vi "SPI API - SPI Simulation.vi"() -> ()   [LabVIEW 2015]
uses:
  Controls/Timing Characteristics.ctl
  Controls/Digital Data.ctl
  <vilib>/rvi/DesktopExecutionNode/Execution/niFpgaDEN_Execute.vi
  <vilib>/rvi/DesktopExecutionNode/DesktopExecutionNode.xnode
panel:
  out "Data 8":u64
  out "Data 7":u64
  out "Data 6":u64
  out "Data 5":u64
  out "Slave Response":u64
  out "Data To Slave":u64 format="%b"
  out "Timing Characteristics":T1 {"tCL (ns)" format="%#_4g"; "tCH (ns)" format="%#_4g"; "tCP (ns)" format="%#_4g"; "tCSS (ns)" format="%#_4g"; "tCSH (ns)" format="%#_4g"; "tCSW (ns)" format="%#_4g"; "Actual Sample Rate (Hz)" format="%_4p"; "SCLK Frequency (Hz)" format="%#.2p"}
  in  "Pause":bool
  in  "SPI PHY Settings":T2={"Divide Value"=10, "Transfer Length (bits)"=24, "CS Asserted Polarity"=FALSE, "Clock Polarity (CPOL)"=FALSE, "Clock Phase (CPHA)"=FALSE, "Lengthen MISO Setup"=FALSE, "Direction Change Bit"=0, "MOSI Starts as Output"=FALSE, "Tristatable MOSI"=FALSE}
  out "Digital Data":digitalwaveform(graph)
  in  "Data To Slave":u64
  in  "Stop":bool
  # "Operating Instructions\n1. For this VI to work, the FPGA must be in Simulation Mode.\n2. Run the VI and change the 'SPI PHY Settings' and 'Data To Slave' controls to change the SPI Output.\n3. While changing the settings, view the timing characteristics of the signal on the right side of the graph."
  # "Typical Timing Diagram"
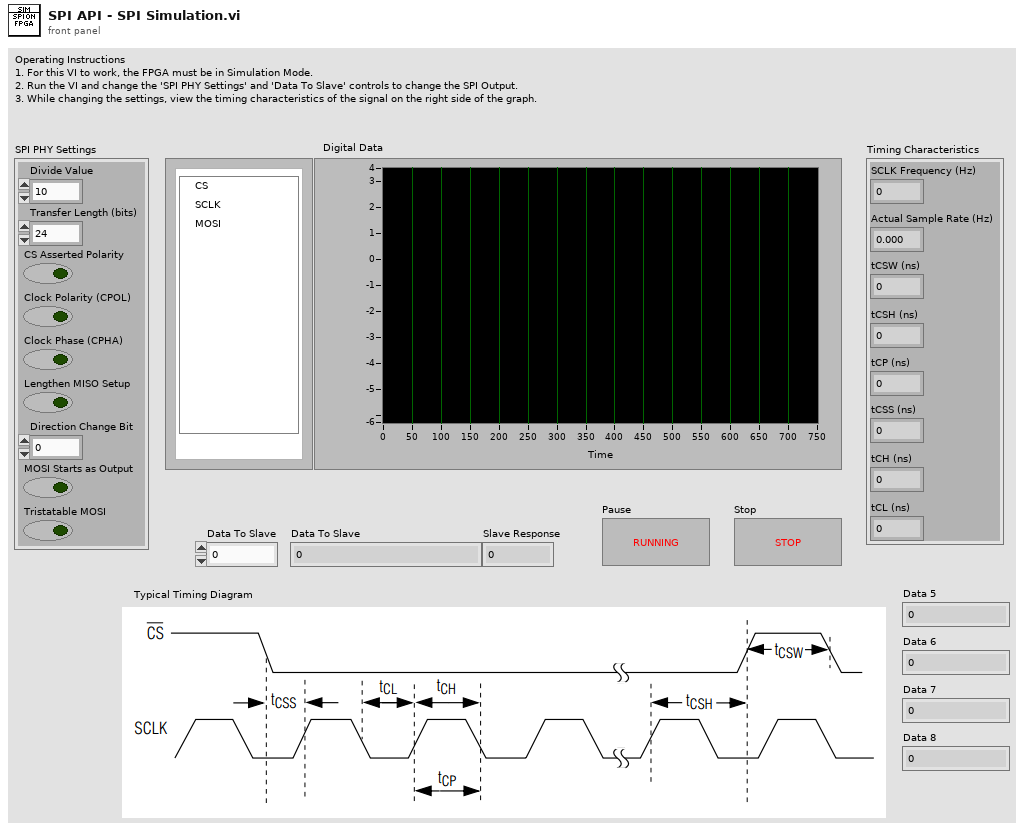
[diagram p1: front panel]
types:
  T1 = typedef "Timing Characteristics.ctl" = cluster{"SCLK Frequency (Hz)":dbl, "Actual Sample Rate (Hz)":dbl, "tCSW (ns)":dbl, "tCSH (ns)":dbl, "tCSS (ns)":dbl, "tCP (ns)":dbl, "tCH (ns)":dbl, "tCL (ns)":dbl}
  T2 = cluster{"Divide Value":u8, "Transfer Length (bits)":u8, "CS Asserted Polarity":bool, "Clock Polarity (CPOL)":bool, "Clock Phase (CPHA)":bool, "Lengthen MISO Setup":bool, "Direction Change Bit":u8, "MOSI Starts as Output":bool, "Tristatable MOSI":bool}
  T3 = typedef "Digital Data.ctl" = cluster{"CS":bool, "SCLK":bool, "MOSI":bool}
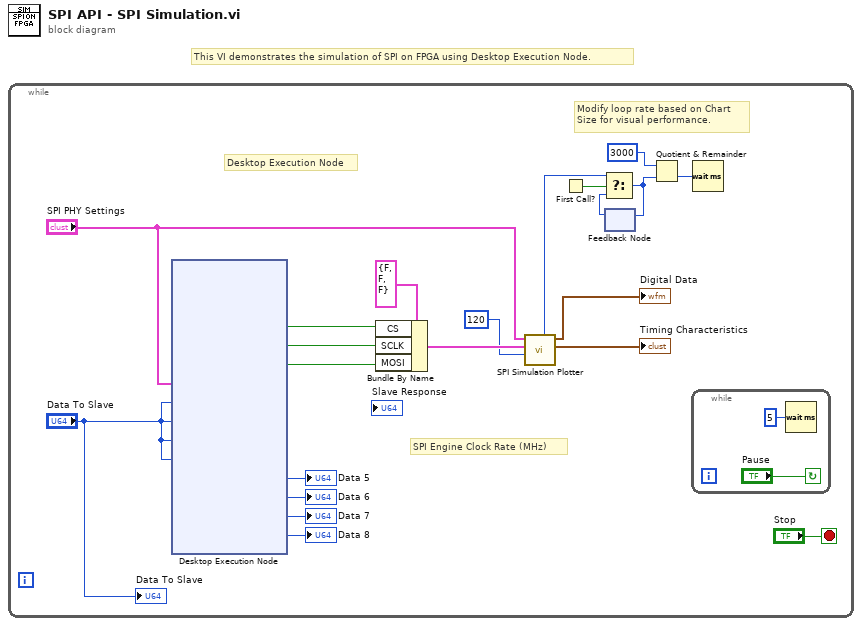
[diagram p0: block diagram]
diagram:
  # "This VI demonstrates the simulation of SPI on FPGA using Desktop Execution Node."
  n1 = while {
    stop <- "Stop" stop-if-true
    # "Desktop Execution Node"
    # "SPI Engine Clock Rate (MHz)"
    # "Modify loop rate based on Chart\nSize for visual performance."
    n2 = xnode "Desktop Execution Node"("SPI Physical Settings"="SPI PHY Settings", "Data 1"="Data To Slave", "Data 2"="Data To Slave", "Data 3"="Data To Slave", "Data 4"="Data To Slave") -> ("CS"=w7:bool, "SCLK"=w8:bool, "MOSI"=w9:bool, "Data 5"=→"Data 5":u64, "Data 6"=→"Data 6":u64, "Data 7"=→"Data 7":u64, "Data 8"=→"Data 8":u64)  [unwired: 1 in, 1 out]
    n3 = Bundle By Name(cluster=T3 {"CS"=FALSE, "SCLK"=FALSE, "MOSI"=FALSE}, "CS"=w7, "SCLK"=w8, "MOSI"=w9) -> (w14:T3)
    n4 = call "SPI Simulation Plotter.vi"("Engine Clock Rate (MHz)"=120, "SPI Signals"=w14, "SPI PHY Settings"="SPI PHY Settings") -> ("Timing Characteristics"=→"Timing Characteristics":T1, "Digital Data"=→"Digital Data":digitalwaveform, "Chart Size"=w13:i32)  [unwired: 6 in]
    n5 = First Call?() -> (First Call?: T/F=w19:bool)
    n6 = feedback #1() -> (w18:i32)  [unwired: 1 in]
    n7 = Select(t=w13, s=w19, f=w18) -> (s? t:f=w17:i32)
    n8 = feedback-in #1(w17) -> ()
    n9 = Quotient & Remainder(x=u32 3000 ("ms per Command"), y=w17) -> (floor(x/y)=w15:u32)  [unwired: 1 out]
    n10 = while {
      stop <- "Pause" continue-if-true
      n11 = Wait (ms)(milliseconds to wait=u32 5) -> ()  [unwired: 1 out]
    }
    n12 = Wait (ms)(milliseconds to wait=w15) -> ()  [unwired: 1 out]
    "Data To Slave" <- "Data To Slave"
  }
